vi "Logistic Random.vi"(6 "seed":i32=-1, 7 "reset":bool, 9 "b":dbl=1.0, 10 "a":dbl, 11 "samples":i32=128) -> (0 "error":i32, 3 "logistic random data":dbl[](array[numeric]))   [LabVIEW 2014, in "NI_Gmath.lvlib"]
doc: "Generates random values from a variate X, where X describes the selected distribution type. You must manually select the polymorphic instance to use."
uses:
  NI_Gmath.lvlib
  st_error_code.ctl
panel:
  # "Logistic Random"
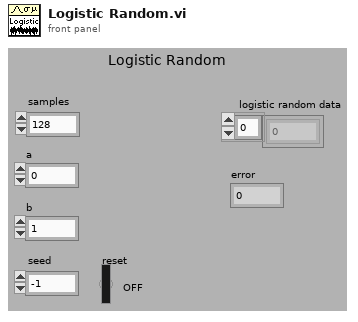
[diagram p1: front panel]
types:
  T1 = typedef "NI_Gmath.lvlib/st_error_code.ctl" = i32
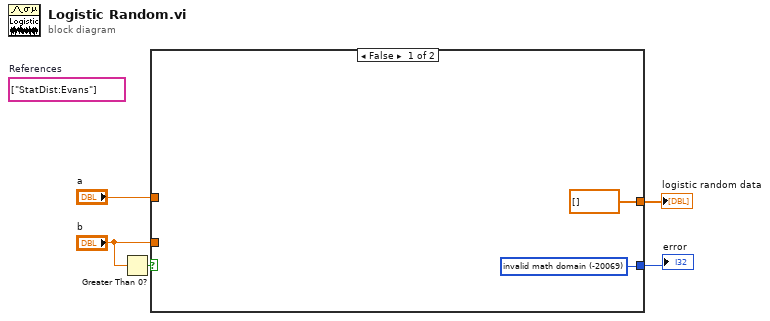
[diagram p0: block diagram]
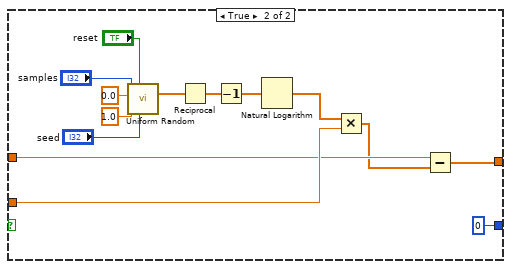
[diagram p2: hidden frame]
diagram:
  (unwired) string[] ["StatDist:Evans"]  # References
  n1 = Greater Than 0?(x="b") -> (x > 0?=w3:bool)
  n2 = case shown="False" w3 {
    tunnel: "b" -> [_ w18]
    tunnel: [w7 0 ("invalid math domain")] -> w1
    tunnel: [dbl[] [] w15] -> w2
    tunnel: "a" -> [_ w16]
    frame False {
      w7 = T1 -20069 items=["invalid math domain"=-20069, "Fourier interpolation size m >= n"=-20070, "empty array"=-20003] ("stat interp error code")
    }
    frame True {
      n3 = call "Uniform Random.vi"("seed"="seed", "reset"="reset", "xmax"=1.0, "xmin"=0.0, "samples"="samples") -> ("uniform random data"=w8:dbl[])  [unwired: 5 in, 1 out]
      n4 = Reciprocal(x=w8) -> (1/x=w20:dbl[])
      n5 = Decrement(x=w20) -> (x-1=w19:dbl[])
      n6 = Natural Logarithm(1:w19) -> (0:w17:dbl[])
      n7 = Multiply(x=w17, y=w18) -> (x*y=w14:dbl[])
      n8 = Subtract(x=w16, y=w14) -> (x-y=w15:dbl[])
    }
  }
  "error" <- w1
  "logistic random data" <- w2
